vi "SetLocalSpec.vi"(8 "error in (no error)":errorcluster, 10 "Path":path, 11 "reference in":refnum<class "MES_Base.lvclass">) -> (0 "error out":errorcluster, 3 "reference in":refnum<class "MES_Base.lvclass">)   [LabVIEW 2022 SP3, in "MES_Base.lvlib" / "MES_Base.lvclass"]
uses:
  MES_Base.lvclass
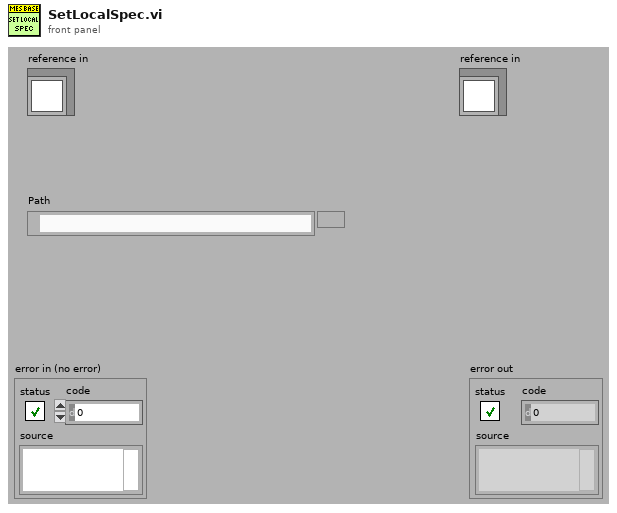
[diagram p1: front panel]
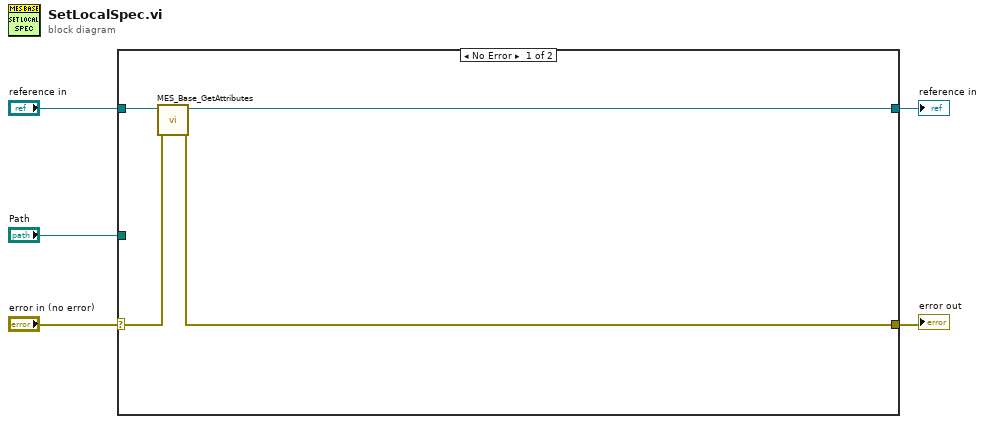
[diagram p0: block diagram]
diagram:
  n1 = case shown="No Error" "error in (no error)" {
    selector: "error in (no error)" -> [w9 w11]
    tunnel: [w8 w11] -> w4
    tunnel: [w6 w10] -> w2
    tunnel: "reference in" -> [w7 w10]
    tunnel: "Path" -> [_ _]
    frame No Error {
      n2 = call "MES_Base_GetAttributes.vi"("error in (no error)"=w9, "reference in"=w7) -> ("error out"=w8:errorcluster, "reference out"=w6:refnum<class "MES_Base.lvclass">)  [unwired: 6 in, 2 out]
    }
    frame Error {
    }
  }
  "error out" <- w4
  "reference in" <- w2
